vi "Init.vi"(8 "error in (no error)":errorcluster, 10 "Topic":string, 11 "AF MQTT Message Channel in":refnum<class "AF MQTT Message Channel.lvclass">) -> (0 "error out":errorcluster, 3 "AF MQTT Message Channel out":refnum<class "AF MQTT Message Channel.lvclass">)   [LabVIEW 2020, in "AF MQTT Channel.lvlib" / "AF MQTT Message Channel.lvclass"]
uses:
  AF MQTT Message Channel.lvclass
  AF MQTT Message Channel.lvclass/AF MQTT Message Channel.ctl
  <vilib>/LabVIEW Open Source Project/MQTT Client/Client class/Client.lvclass
  C:/Program Files (x86)/National Instruments/LabVIEW 2020/vi.lib/LabVIEW Open Source Project/MQTT Connection/MQTT_Base/Base Class/MQTT_Base.lvclass
  Actor Pub Sub Channels/Pub Sub Message Channel/Pub Sub Message Channel.lvclass
  <vilib>/LabVIEW Open Source Project/MQTT Connection/MQTT_Base/Base Class/MQTT_Base.lvclass
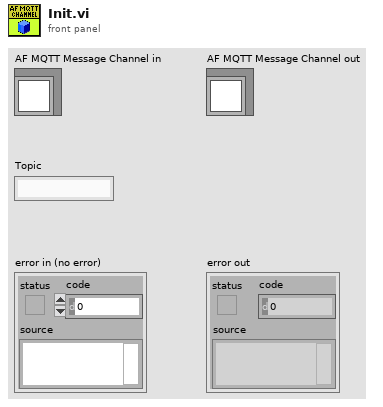
[diagram p1: front panel]
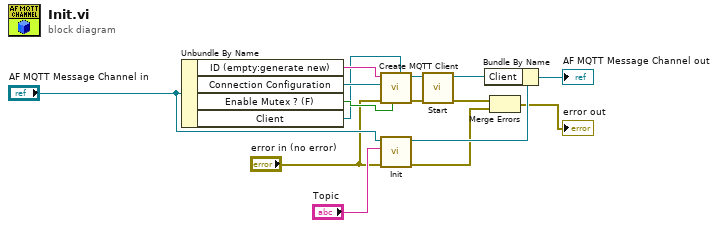
[diagram p0: block diagram]
diagram:
  n1 = Unbundle By Name("AF MQTT Message Channel in") -> ("ID (empty:generate new)"=w12:string, "Connection Configuration"=w11:refnum<class "Connection.lvclass">, "Enable Mutex ? (F)"=w10:bool, "Client"=w8:refnum<class "Client.lvclass">)
  n2 = call <vilib>:"Create MQTT Client.vi"("Client in"=w8, "Enable Mutex ? (F)"=w10, "error in (no error)"="error in (no error)", "Connection Configuration"=w11, "ID (empty:generate new)"=w12) -> ("error out"=w2:errorcluster, "Client out"=w4:refnum<class "Client.lvclass">)  [unwired: 5 in]
  n3 = call-parent "Init.vi"("error in (no error)"="error in (no error)", "Topic"="Topic", "Pub Sub Message Channel in"="AF MQTT Message Channel in") -> ("error out"=w5:errorcluster, "Pub Sub Message Channel out"=w15:refnum<class "AF MQTT Message Channel.lvclass">)  [unwired: 7 in]
  n4 = call <vilib>:"Start.vi"("error in (no error)"=w2, "MQTT_Base in"=w4) -> ("error out"=w1:errorcluster, "MQTT_Base out"=w3:refnum<class "Client.lvclass">)  [unwired: 7 in, 1 out]
  n5 = Bundle By Name(cluster=w15, "Client"=w3) -> (→"AF MQTT Message Channel out":refnum<class "AF MQTT Message Channel.lvclass">)
  n6 = Merge Errors(w1, w5) -> (→"error out":errorcluster)
